vi "Read NewValue.vi"(8 "error in (no error)":errorcluster, 11 "MetaDriver_v1 in":refnum<class "MetaDriver_v1.lvclass">) -> (0 "error out":errorcluster, 2 "NewValue":variant, 3 "MetaDriver_v1 out":refnum<class "MetaDriver_v1.lvclass">)   [LabVIEW 2020, in "MetaDriver_v1.lvclass"]
uses:
  MetaDriver_v1.lvclass
  MetaDriver_v1.lvclass/MetaDriver_v1.ctl
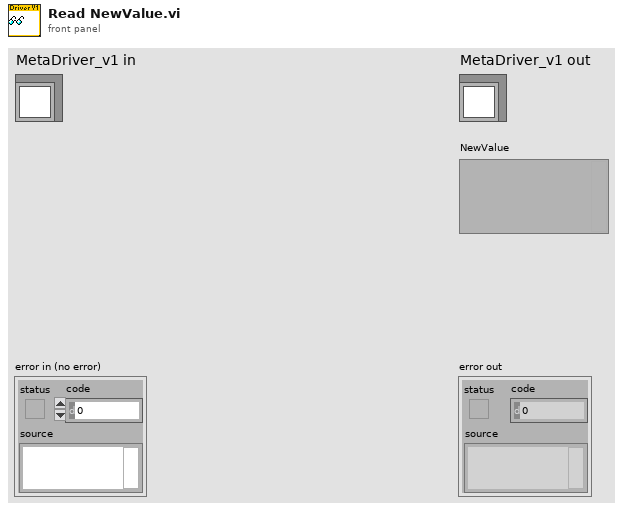
[diagram p1: front panel]
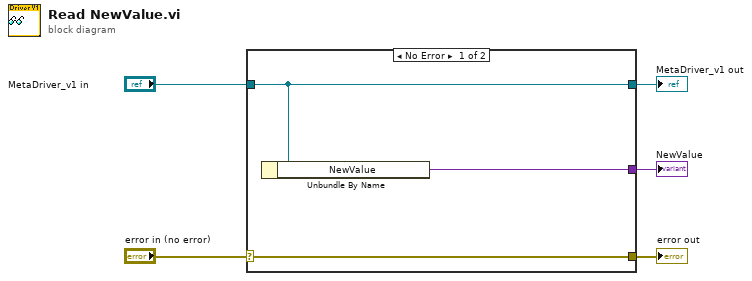
[diagram p0: block diagram]
diagram:
  n1 = case shown="No Error" "error in (no error)" {
    selector: "error in (no error)" -> [w8 w9]
    tunnel: [w8 w9] -> w4
    tunnel: [w7 w10] -> w2
    tunnel: "MetaDriver_v1 in" -> [w7 w10]
    tunnel: [w6 _] -> w1
    frame No Error {
      n2 = Unbundle By Name(w7) -> ("NewValue"=w6:variant)
    }
    frame Error {
    }
  }
  "error out" <- w4
  "MetaDriver_v1 out" <- w2
  "NewValue" <- w1
